vi "Format File Entry.vi"(8 "error in (no error)":errorcluster, 11 "message":string) -> (0 "error out":errorcluster, 3 "formatted string":string)   [LabVIEW 2021, in "Diagnostics.lvlib"]
uses:
  Diagnostics.lvlib
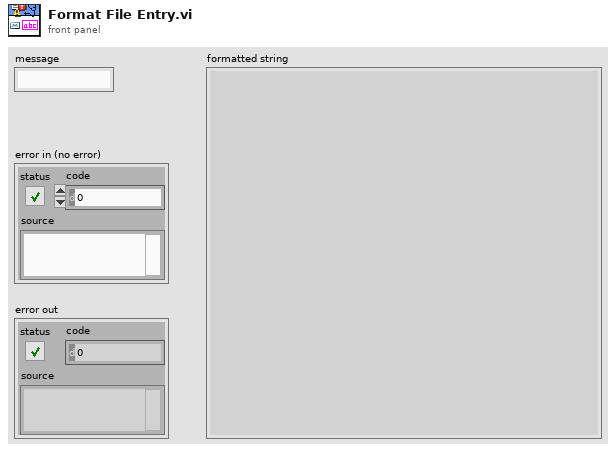
[diagram p1: front panel]
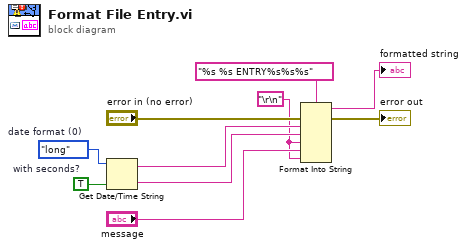
[diagram p0: block diagram]
diagram:
  w1 = enum16{"short", "long", "abbreviated"}."long"  # date format (0)
  w2 = TRUE  # with seconds?
  w3 = "\r\n"
  n1 = Get Date/Time String(date format (0)=w1, want seconds? (F)=w2) -> (date string=w5:string, time string=w6:string)  [unwired: 1 in]
  n2 = Format Into String(format string="%s %s ENTRY%s%s%s", error in="error in (no error)", w5, w6, w3, "message", w3) -> (resulting string=→"formatted string":string, error out=→"error out":errorcluster)  [unwired: 1 in]
